vi "Read LVCluster Pointer by Para.vi"() -> ()   [LabVIEW 2012]
uses:
  demo dll.dll
panel:
  out "LVCluster":cluster{"U8":u8, "I32":i32, "DBL":dbl}
  in  "Pack1Cluster":cluster{"U8":u8, "I32":i32, "DBL":dbl}
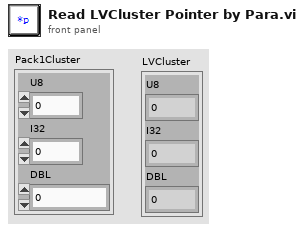
[diagram p1: front panel]
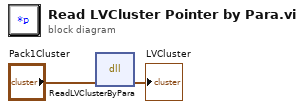
[diagram p0: block diagram]
diagram:
  n1 = dll-call lib="PTH1+abs EBOOK\t功能块DLLdemo dll.dll" fn="ReadLVClusterByPara"("LVCluster"="Pack1Cluster") -> ("LVCluster"=→"LVCluster":cluster{"U8":u8, "I32":i32, "DBL":dbl})  [unwired: 4 in, 2 out]
